vi "Create.vi"   [LabVIEW 2020, in "feature_detection.lvlib" / "Text Detector.lvclass"]
uses:
  Text Detector.lvclass
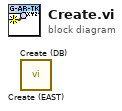
[diagram p0: block diagram]
diagram:
  n1 = call "Create (EAST).vi"() -> ()  [unwired: 10 in, 2 out]
  n2 = call "Create (DB).vi"() -> ()  [unwired: 10 in, 2 out]
